vi "Map Viewer.vi"() -> ()   [LabVIEW 2012]
panel:
  in  "stop":bool
  out "Intensity Graph":dbl[][](graph)
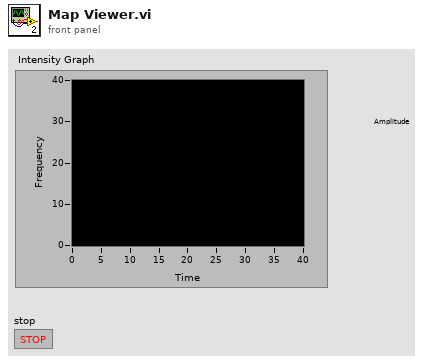
[diagram p1: front panel]
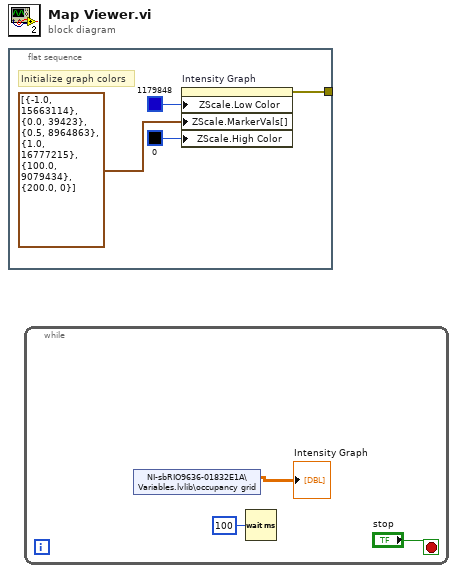
[diagram p0: block diagram]
diagram:
  n1 = flat-sequence {
    tunnel: [w1] -> _
    frame #0 {
      # "Initialize graph colors"
      n2 = property on="Intensity Graph" class="IntGraph (strict)"("ZScale.Low Color"=u32 1179848, "ZScale.MarkerVals[]"=cluster{dbl, u32}[] [{-1.0, 15663114}, {0.0, 39423}, {0.5, 8964863}, {1.0, 16777215}, {100.0, 9079434}, {200.0, 0}], "ZScale.High Color"=u32 0) -> (error out=w1:errorcluster)  [unwired: 2 in, 1 out]
    }
  }
  n3 = while {
    stop <- "stop" stop-if-true
    n4 = shared-variable "NI-sbRIO9636-01832E1A\\Variables.lvlib\\occupancy grid"() -> (→"Intensity Graph":dbl[][])  [unwired: 1 in, 1 out]
    n5 = Wait (ms)(milliseconds to wait=u32 100) -> ()  [unwired: 1 out]
  }
